vi "Read Virt Instr CFG.vi"(8 "error in":errorcluster, 10 "Virt Instr CFG":path, 11 "File Provider in":refnum<class "File Provider.lvclass">) -> (0 "error out":errorcluster, 3 "File Provider out":refnum<class "File Provider.lvclass">)   [LabVIEW 2023, in "File Provider.lvlib" / "File Provider.lvclass"]
uses:
  File Provider.lvclass
  File Provider.lvclass/File Provider.ctl
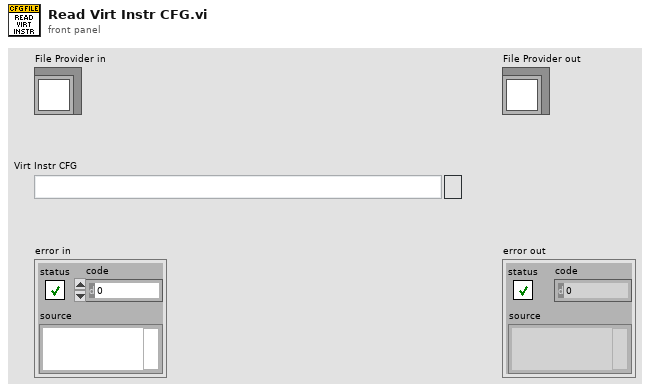
[diagram p1: front panel]
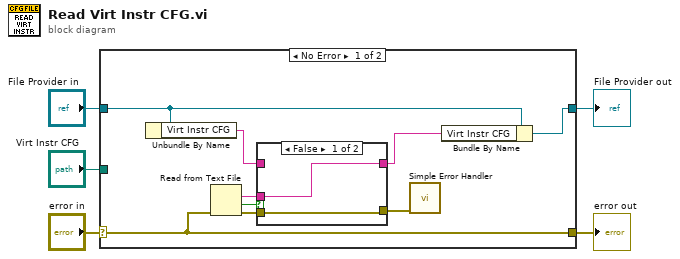
[diagram p0: block diagram]
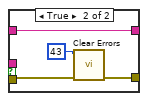
[diagram p2: hidden frame]
diagram:
  n1 = case shown="No Error" "error in" {
    selector: "error in" -> [w14 w22]
    tunnel: [w14 w22] -> w4
    tunnel: [w8 w21] -> w2
    tunnel: "File Provider in" -> [w9 w21]
    tunnel: "Virt Instr CFG" -> [_ _]
    frame No Error {
      n2 = Unbundle By Name(w9) -> ("Virt Instr CFG"=w10:string)
      n3 = Read from Text File(error in=w14) -> (text=w11:string, cancelled=w13:bool, error out=w12:errorcluster)  [unwired: 3 in, 1 out]
      n4 = case shown="False" w13 {
        tunnel: w12 -> [w15 w19]
        tunnel: w11 -> [w16 _]
        tunnel: w10 -> [_ w20]
        tunnel: [w16 w20] -> w7
        tunnel: [w15 w17] -> w6
        frame False {
        }
        frame True {
          n5 = call <vilib>:"Clear Errors.vi"("error in (no error)"=w19, "specific error code to clear (0: all)"=43) -> ("error out"=w17:errorcluster)  [unwired: 4 in, 1 out]
        }
      }
      n6 = call <vilib>:"Simple Error Handler.vi"("error in (no error)"=w6) -> ()  [unwired: 4 in, 5 out]
      n7 = Bundle By Name(cluster=w9, "Virt Instr CFG"=w7) -> (w8:refnum<class "File Provider.lvclass">)
    }
    frame Error {
    }
  }
  "error out" <- w4
  "File Provider out" <- w2
